vi "Remote_Gas_desk_Control.vi"(3 "Mode":T5, 5 "Traverse line In":T2 {"Row Duration (mins)" format="%#.1f"; "Row No" min=0; "Trace Gas Concentration (%)" min=0.0 format="%#.2f"; "Emission Rate (l/min)" format="%#.2f"; "Tunnel Speed" format="%#.2f"; "Start X" format="%#.2f"; "Start Y" format="%#.2f"; "Start Z" format="%#.2f"; "End X" format="%#.2f"; "End Y" format="%#.2f"; "End Z" format="%#.2f"; "Averaging time (min)" min=0.0 format="%#.1f"}) -> (0 "Error Message":string, 1 "Status":T1, 2 "Traverse line Out":T2 {"Row Duration (mins)" format="%#.1f"; "Row No" min=0; "Trace Gas Concentration (%)" min=0.0 format="%#.2f"; "Emission Rate (l/min)" format="%#.2f"; "Tunnel Speed" format="%#.2f"; "Start X" format="%#.2f"; "Start Y" format="%#.2f"; "Start Z" format="%#.2f"; "End X" format="%#.2f"; "End Y" format="%#.2f"; "End Z" format="%#.2f"; "Averaging time (min)" min=0.0 format="%#.1f"})   [LabVIEW 2010]
uses:
  Gen Trav/Multi_Run_Status.ctl
  Controls/Stack_release.ctl
  ADAM Client/Sub VIs/ADAM Controls/Client_Source_Status.ctl
  Controls/User_Specific_mode.ctl
  Controls/Post_Process.ctl
  Gen Trav/Spacing.ctl
  Gen Trav/Traverse_cluster.ctl
  Controls/Multi_run_mode.ctl
panel:
  # "X           Y            Z"
  # "Start"
  # "End"
  # "X           Y            Z"
  # "Start"
  # "End"
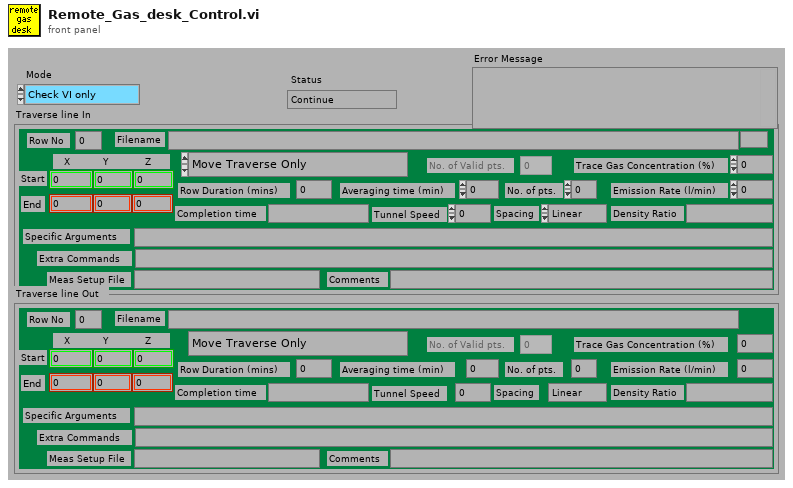
[diagram p1: front panel]
types:
  T1 = typedef "Multi_Run_Status.ctl" = enum16{"Continue", "Jump to Next Point", "Jump to Next Row", "Jump To Fall Back", "Terminate Run"}
  T2 = typedef "Traverse_cluster.ctl" = cluster{"Start X":dbl, "Start Y":dbl, "Start Z":dbl, "End X":dbl, "End Y":dbl, "End Z":dbl, "No. of pts.":i32, "Spacing":T3, "Filename":path, "Tunnel Speed":dbl, "Averaging time (min)":dbl, "Extra Commands":string, "Specific Arguments":string, "Emission Rate (l/min)":dbl, "Trace Gas Concentration (%)":dbl, "Density Ratio":string, "Comments":string, "Row No":i32, "Row Type Selector":T4, "Completion time":string, "Row Duration (mins)":dbl, "No. of Valid pts.":i32, "Meas Setup File":string}
  T3 = typedef "Spacing.ctl" = enum16{"Linear", "Log", "Gauss", "Specified", "N/A"}
  T4 = typedef "Multi_run_mode.ctl" = enum16{"Move Traverse Only", "Set Tunnel Speed Only", "Set Source Only", "Set Measurement Conditions", "Single Measurement", "Vertical Profile", "Lateral Profile", "Longitudinal Profile", "Explore Volume", "Multi-Axis Profile", "Auto Calibrate", "Meas Fast FID Bkgnd", "Check Beam Power", "Scanning Valve Measurement", "Run VI Named:", "Set ADAM Ch", "Wait (minutes)", "Send Message", "Synchronize With:", "Fall Back to this Row", "Turn Off Row Repeating", "Blank Row"}
  T5 = typedef "User_Specific_mode.ctl" = enum16{"Check VI only", "Run VI"}
  T6 = typedef "Client_Source_Status.ctl" = enum16{"Not Using", "Using", "Must Have"}
  T7 = typedef "Post_Process.ctl" = enum16{"Take New Data", "Post Process Raw Data File"}
  T8 = typedef "Stack_release.ctl" = enum16{"Fill and Analyse Coils", "Just Analyse Coils"}
  T9 = enum16{"Run Program", "Save Current Setup", "Setup front panel"}
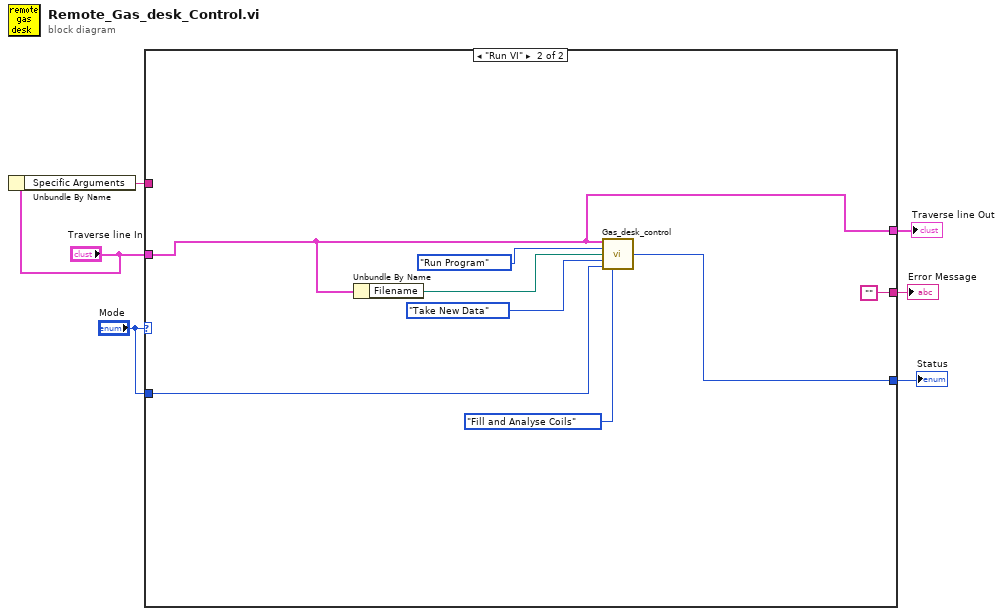
[diagram p0: block diagram]
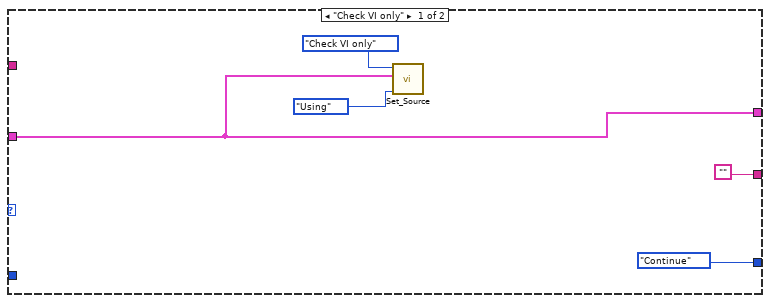
[diagram p2: hidden frame]
diagram:
  n1 = Unbundle By Name("Traverse line In") -> ("Specific Arguments"=w3:string)
  n2 = case shown="\"Run VI\"" "Mode" {
    tunnel: ["" ""] -> w6
    tunnel: "Traverse line In" -> [w7 w14]
    tunnel: [w7 w14] -> w5
    tunnel: w3 -> [_ _]
    tunnel: [Multi_Run_Status."Continue" ("Status") w17] -> w2
    tunnel: "Mode" -> [_ w16]
    frame "Check VI only" {
      n3 = call "Set_Source.vi"("Source Status"=Client_Source_Status."Using", "Traverse line"=w7, "Simulate/Run"=User_Specific_mode."Check VI only") -> ()  [unwired: 1 in, 6 out]
    }
    frame "Run VI" {
      n4 = Unbundle By Name(w14) -> ("Filename"=w13:path)
      n5 = call "Gas_desk_control.vi"("Traverse line"=w14, "setup"=T9."Run Program", "Results File"=w13, "Post Process"=Post_Process."Take New Data", "Simulate/Run"=w16, "Release control"=Stack_release."Fill and Analyse Coils") -> ("Status"=w17:T1)  [unwired: 9 in]
    }
  }
  "Error Message" <- w6
  "Traverse line Out" <- w5
  "Status" <- w2
